vi "Pre Launch Init.vi"(11 "MediatorBusMonitor in":refnum<class "MediatorBusMonitor.lvclass">) -> (0 "error out":errorcluster, 3 "MediatorBusMonitor out":refnum<class "MediatorBusMonitor.lvclass">)   [LabVIEW 2017, in "Mediator.lvlib" / "MediatorBusMonitor.lvclass"]
doc: "(<B>Filename</B>: Actor Framework.lvlib:Actor.lvclass:Pre Launch Init.vi)\n\nDefines behavior that occurs after the Launch Nested Actor method is invoked but before the actor's Actor Core method begins running.\n\nBy default, this method does nothing. A descendant class may override it to define behavior."
uses:
  MediatorBusMonitor.lvclass
  C:/Program Files (x86)/National Instruments/LabVIEW 2017/vi.lib/ActorFramework/Actor/Actor.lvclass
  MediatorBusMonitor Messages/Update Front Panel Msg/Update Front Panel Msg.lvclass
  C:/Program Files (x86)/National Instruments/LabVIEW 2017/vi.lib/ActorFramework/Message/Message.lvclass
  MediatorBusMonitor.lvclass/MediatorBusMonitor.ctl
  <vilib>/ActorFramework/Actor/Actor.lvclass/Actor.ctl
  <vilib>/ActorFramework/Message Enqueuer/Message Enqueuer.lvclass/Message Enqueuer.ctl
  gpm_packages/@cs/actor-framework-messages/Source/MessageCycle/MessageCycle.lvclass/MessageCycle.ctl
  <vilib>/ActorFramework/Message Enqueuer/Init from Existing Queue.vi
  <vilib>/ActorFramework/Message Enqueuer/Enqueue.vi
  gpm_packages/@cs/actor-framework-messages/Source/MessageCycle/MessageCycle.lvclass
  <vilib>/ActorFramework/Message Priority Queue/Priority Enqueue.vi
  gpm_packages/@cs/actor-framework-messages/Source/MessageCycle/Launch Deferred Timeout Notifier.vi
  IMediator/IMediatorBusMonitor/MediatorBusMonitor/IMediatorBusMonitor.lvclass
  <vilib>/ActorFramework/Message/Message.lvclass
  <vilib>/ActorFramework/Message Enqueuer/Message Enqueuer.lvclass
  <vilib>/ActorFramework/Actor/Actor.lvclass
  gpm_packages/@cs/lookup-table/Source/LookupTable/LookupTable.lvclass
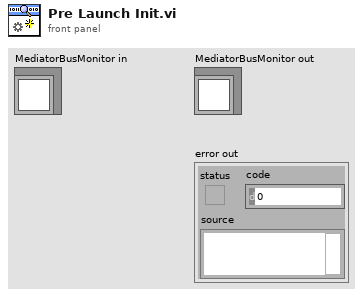
[diagram p1: front panel]
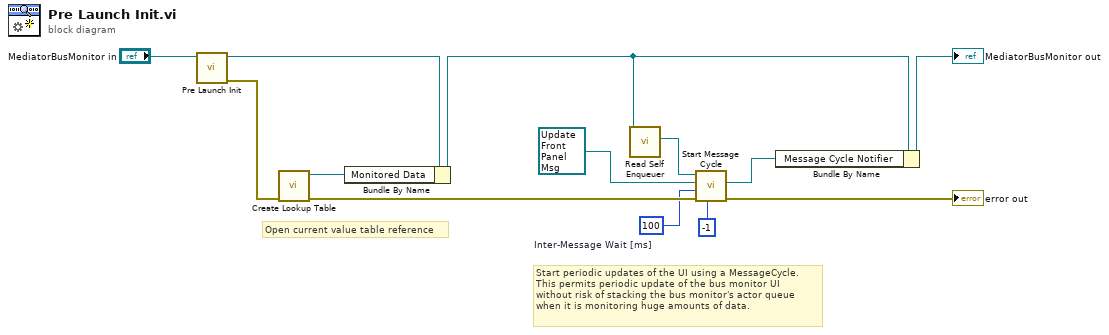
[diagram p0: block diagram]
diagram:
  w1 = 100  # Inter-Message Wait [ms]
  # "Start periodic updates of the UI using a MessageCycle.\nThis permits periodic update of the bus monitor UI\nwithout risk of stacking the bus monitor's actor queue\nwhen it is monitoring huge amounts of data."
  # "Open current value table reference"
  n1 = call-parent "Pre Launch Init.vi"("IViewable in"="MediatorBusMonitor in") -> ("error out"=w10:errorcluster, "IViewable out"=w13:refnum<class "MediatorBusMonitor.lvclass">)  [unwired: 9 in]
  n2 = call "Create Lookup Table.vi"("error in (no error)"=w10) -> ("error out"=w9:errorcluster, "LookupTable Reference"=w11:refnum<data-value>)  [unwired: 9 in]
  n3 = Bundle By Name(cluster=w13, "Monitored Data"=w11) -> (w7:refnum<class "MediatorBusMonitor.lvclass">)
  n4 = call <vilib>:"Read Self Enqueuer.vi"("Actor"=w7) -> ("Self Enqueuer"=w6:refnum<class "Message Enqueuer.lvclass">)  [unwired: 10 in]
  n5 = call "Start Message Cycle.vi"("Cycle Timeout [ms] (-1)"=-1, "error in (no error)"=w9, "Inter-Message Wait [ms] (0)"=w1, "Message"=refnum<class "Update Front Panel Msg.lvclass"> refnum ("Mediator.lvlib:Update Front Panel Msg.lvclass"), "Message Enqueuer"=w6) -> ("error out"=→"error out":errorcluster, "Message Cycle Notifier"=w2:refnum<notifier>)  [unwired: 4 in, 1 out]
  n6 = Bundle By Name(cluster=w7, "Message Cycle Notifier"=w2) -> (→"MediatorBusMonitor out":refnum<class "MediatorBusMonitor.lvclass">)
